vi "Camera.vi"() -> ()   [LabVIEW 2015]
uses:
  Camera Properties.ctl
  ModeEnum.ctl
  CameraState.ctl
  Stack_State.ctl
  Stack Track.ctl
  CameraControlTypeDef.ctl
  Waveform Generation/WaveformControllerState.ctl
  <vilib>/DAQmx/write.llb/DAQmx Write (Digital 1D Wfm NChan NSamp).vi
  <vilib>/DAQmx/write.llb/DAQmx Write (Analog 1D Wfm NChan NSamp).vi
  <vilib>/DAQmx/create/channels.llb/DAQmx Create Channel (AO-Voltage-Basic).vi
  <vilib>/DAQmx/configure/timing.llb/DAQmx Timing (Sample Clock).vi
  <vilib>/Waveform/DWDTOps.llb/DWDT Uncompress Digital.vi
  <vilib>/DAQmx/miscellaneous.llb/DAQmx Fill In Error Info.vi
  <vilib>/DAQmx/create/channels.llb/DAQmx Create Channel (DO-Digital Output).vi
  <vilib>/vision/NI_Vision_Development_Module.lvlib
panel:
  in  "Tab Control":enum32{"Camera Settings", "Recording"}(tab)
  in  "Camera Mode":T1(ring)
  in  "Slit Width /percent":dbl=100.0
  out "error IO":errorcluster
  in  "V Height":dbl=2048.0 min=4.0 max=2048.0 step=4.0
  in  "V Offset":dbl min=0.0 max=0.0 step=4.0
  in  "H Offset":dbl min=0.0 max=0.0 step=4.0
  in  "H Width":dbl min=4.0 max=2048.0 step=4.0
  in  "Exposure /ms":dbl=40.0 min=0.0010036691729323308 max=10.000004210526315 step=1e-08
  in  "Trigger Source":dbl(ring)=2.0 items=["Internal"=1.0, "External"=2.0]
  in  "Readout Direction":dbl(ring)=2.0 items=["Forward"=1.0, "Backward"=2.0]
  in  "Scanning Mode":dbl(ring)=12.0 items=["Full Frame"=1.0, "Slit Scanning"=12.0]
  in  "Advanced DCAM Controls":i32(listbox) caption="Multicolumn Listbox"
  in  "Mode":T2
  in  "FOV /um":dbl(slide) scale=-10.0..10.0
  in  "Properties":T3=4211904 items=["SENSOR MODE"=4212128, "CCD MODE"=4212384, "READOUT MODE"=4211872, "ACTIVE VIEW INDEX"=4343136, "BITS PER CHANNEL"=4342976, "IMAGE PIXEL TYPE"=4343296, "BINNING"=4215968, "EXPOSURE TIME"=2049184, "CONTRAST GAIN"=3163312, "CONTRAST OFFSET"=3163328, "LIGHT MODE"=2114720, "SENSITIVITY"=2114992, "PHOTON IMAGING MODE"=2115200, "HIGH DYNAMIC RANGE MODE"=3163360, "WHITE BALANCE"=3163568, "TEMPERATURE"=2115232, "TEMPERATURE TARGET"=2115264, "SENSOR COOLER FAN"=2115296, "LINEBUNDLE HEIGHT"=4212192, "MECHANICAL SHUTTER"=2115488, "BACK FOCUS POSITION"=8422304, "TRIGGER CONNECTOR"=1066432, "TRIGGER SOURCE"=1066144, "OUTPUT TRIGGER SOURCE"=1852576, "TRIGGER GLOBAL EXPOSURE"=2049680, "FIRST TRIGGER BEHAVIOR"=2049696, "CHANNEL SYNC"=1852352, "READOUT DIRECTION"=4211904, "PRE HSYNC COUNT"=1852704, "INTERNAL LINE SPEED"=4191408, "INTERNAL LINE INVERVAL"=4191424]
  out "Image":T4(plugin-control)
  out "Histogram":T5(graph)
  in  "stop":bool
  in  "Calibration":bool
  in  "MultiD Scan":bool
  in  "Stage Controller":bool
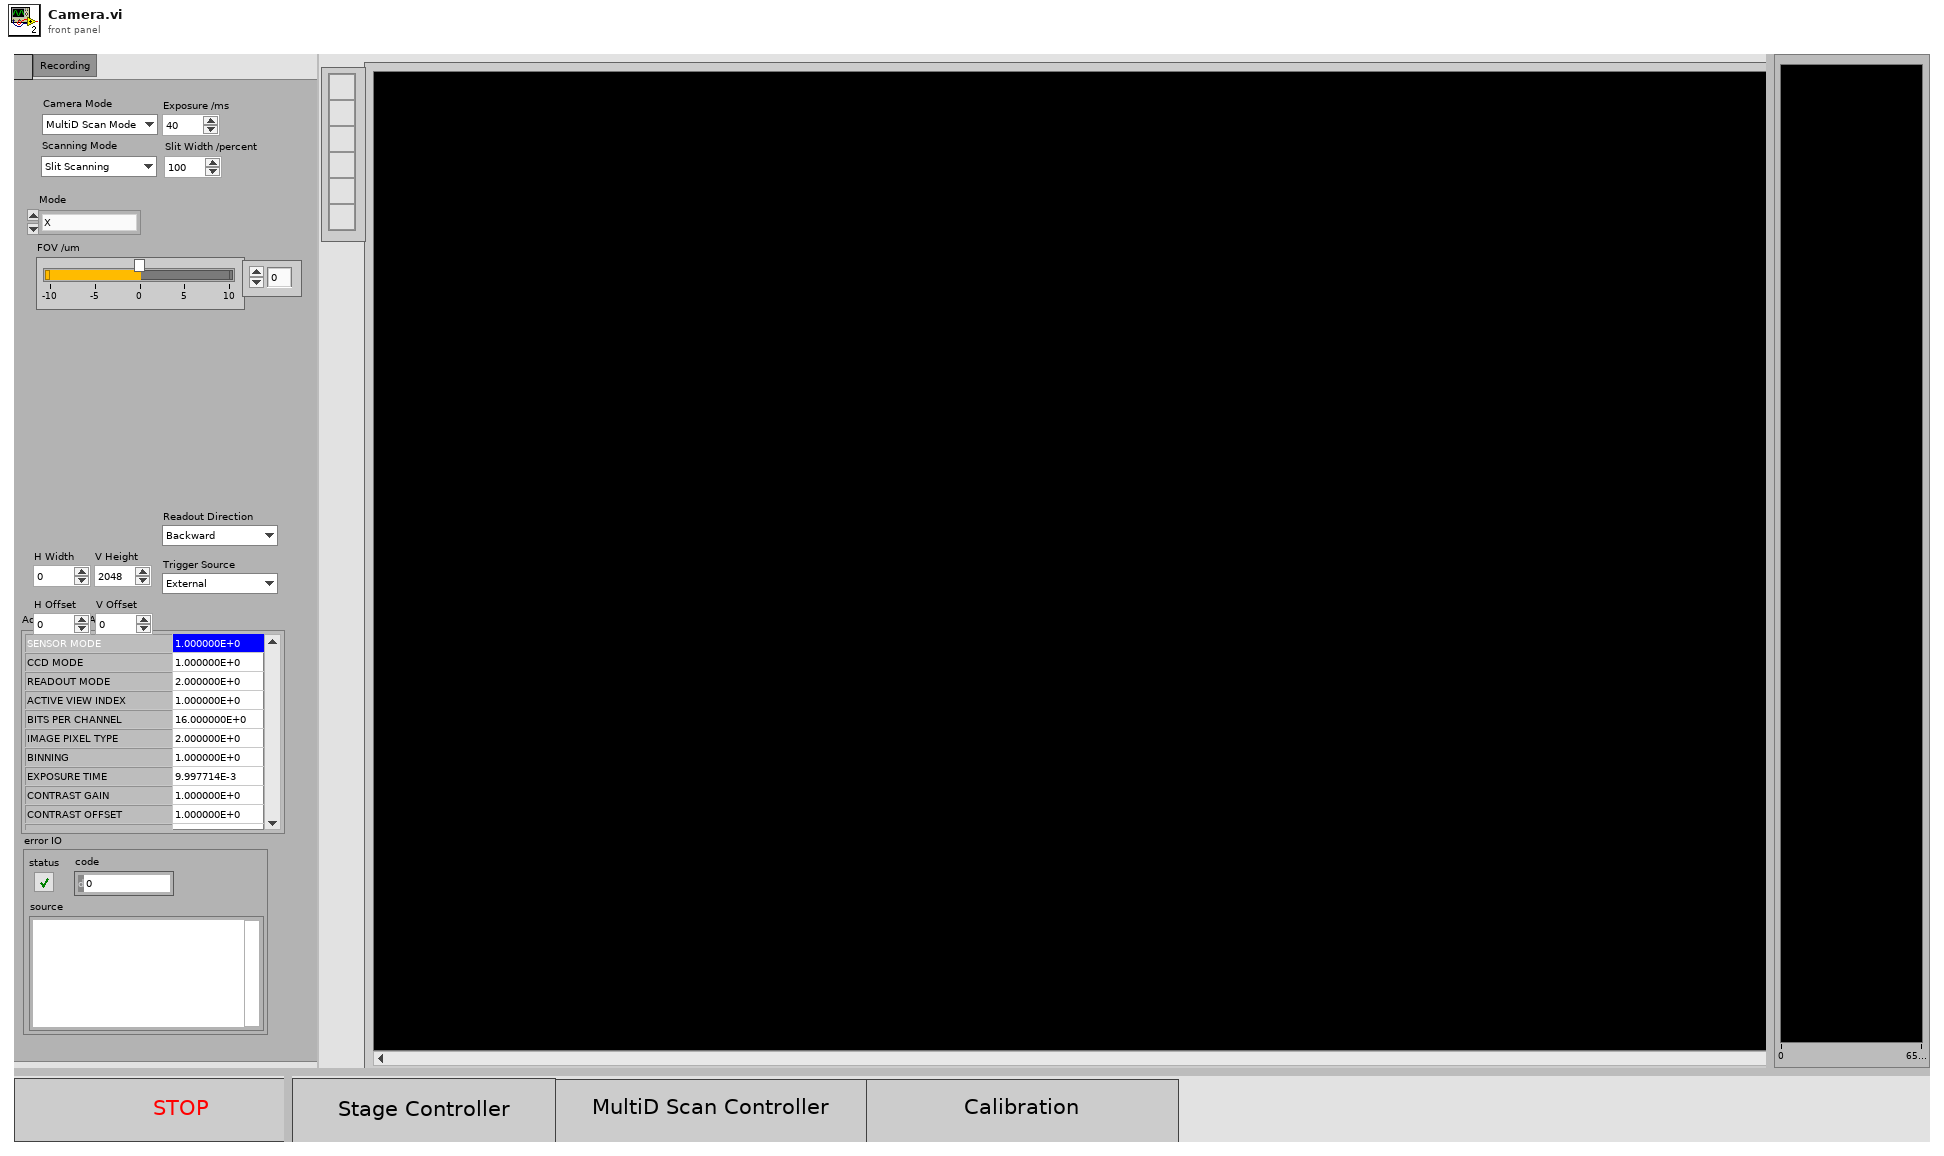
[diagram p1: front panel]
types:
  T1 = enum16{"MultiD Scan Mode", "2D Scan Mode", "Calibration Mode"}
  T2 = typedef "ModeEnum.ctl" = enum16{"X", "XY", "XYZ", "XYZT", "runWaves", "generateWaves", "deInit", "Init", "Idle"}
  T3 = typedef "Camera Properties.ctl" = u32
  T4 = typedef "IMAQ Image.ctl" = refnum<image>
  T5 = cluster{"Starting Value":sgl, "Incremental Value":sgl, "Histogram":u32[]}
  T6 = cluster{"Piezo Position /um":dbl, "Exposure/ms":dbl, "Samples/millisecond":dbl, "Relax/ms":dbl}
  T7 = typedef "WaveformControllerState.ctl" = enum16{"X", "XY", "XYZ", "XYZT", "runWaves", "generateWaves", "deInit", "Init", "Idle"}
  T8 = typedef "CameraControlTypeDef.ctl" = enum16{"IntervalLineInt", "Ram Record", "HardDisk Record", "Disengage Update", "Update", "Idle", "ROI", "Binning", "Scan Mode", "Trigger Mode", "Readout Mode", "Readout Direction", "Preview", "ROIWindow", "Trigger Source"}
  T9 = cluster{"height":u32, "width":u32, "datatype":u32}
  T10 = typedef "Stack_State.ctl" = cluster{"State":T11, "Stack Number":i32, "Image":u16[][], "Stacks":i32}
  T11 = typedef "Stack Track.ctl" = enum16{"Idle", "Display", "Start Sequence", "Read Disk", "STOP", "Collecting", "End"}
  T12 = typedef "CameraState.ctl" = enum16{"init", "active", "deinit"}
  T13 = cluster{T7, cluster{"Piezo Position /um":dbl, "Exposure/ms":dbl, "Samples/millisecond":dbl, "Relax/ms":dbl}}
  T14 = typedef "Image Type" = u32
  T15 = cluster{"Value":i32, "Minimum":i32, "Maximum":i32, "Increment":i32}
  T16 = cluster{"Minimum":i32, "Maximum":i32, "Increment":i32}
  T17 = cluster{"Enum":T8, dbl, "timeout in ms (-1)":u32}
  T18 = cluster{"State":T11, "Timeout":i32, "Data 16":u16[][], "Timeout":i32}
  T19 = cluster{"Enum":T8, "Trigger Source":dbl, "timeout in ms (-1)":i32}
  T20 = cluster{"Enum":T8, "Exposure /ms":dbl, "Parameter":u32}
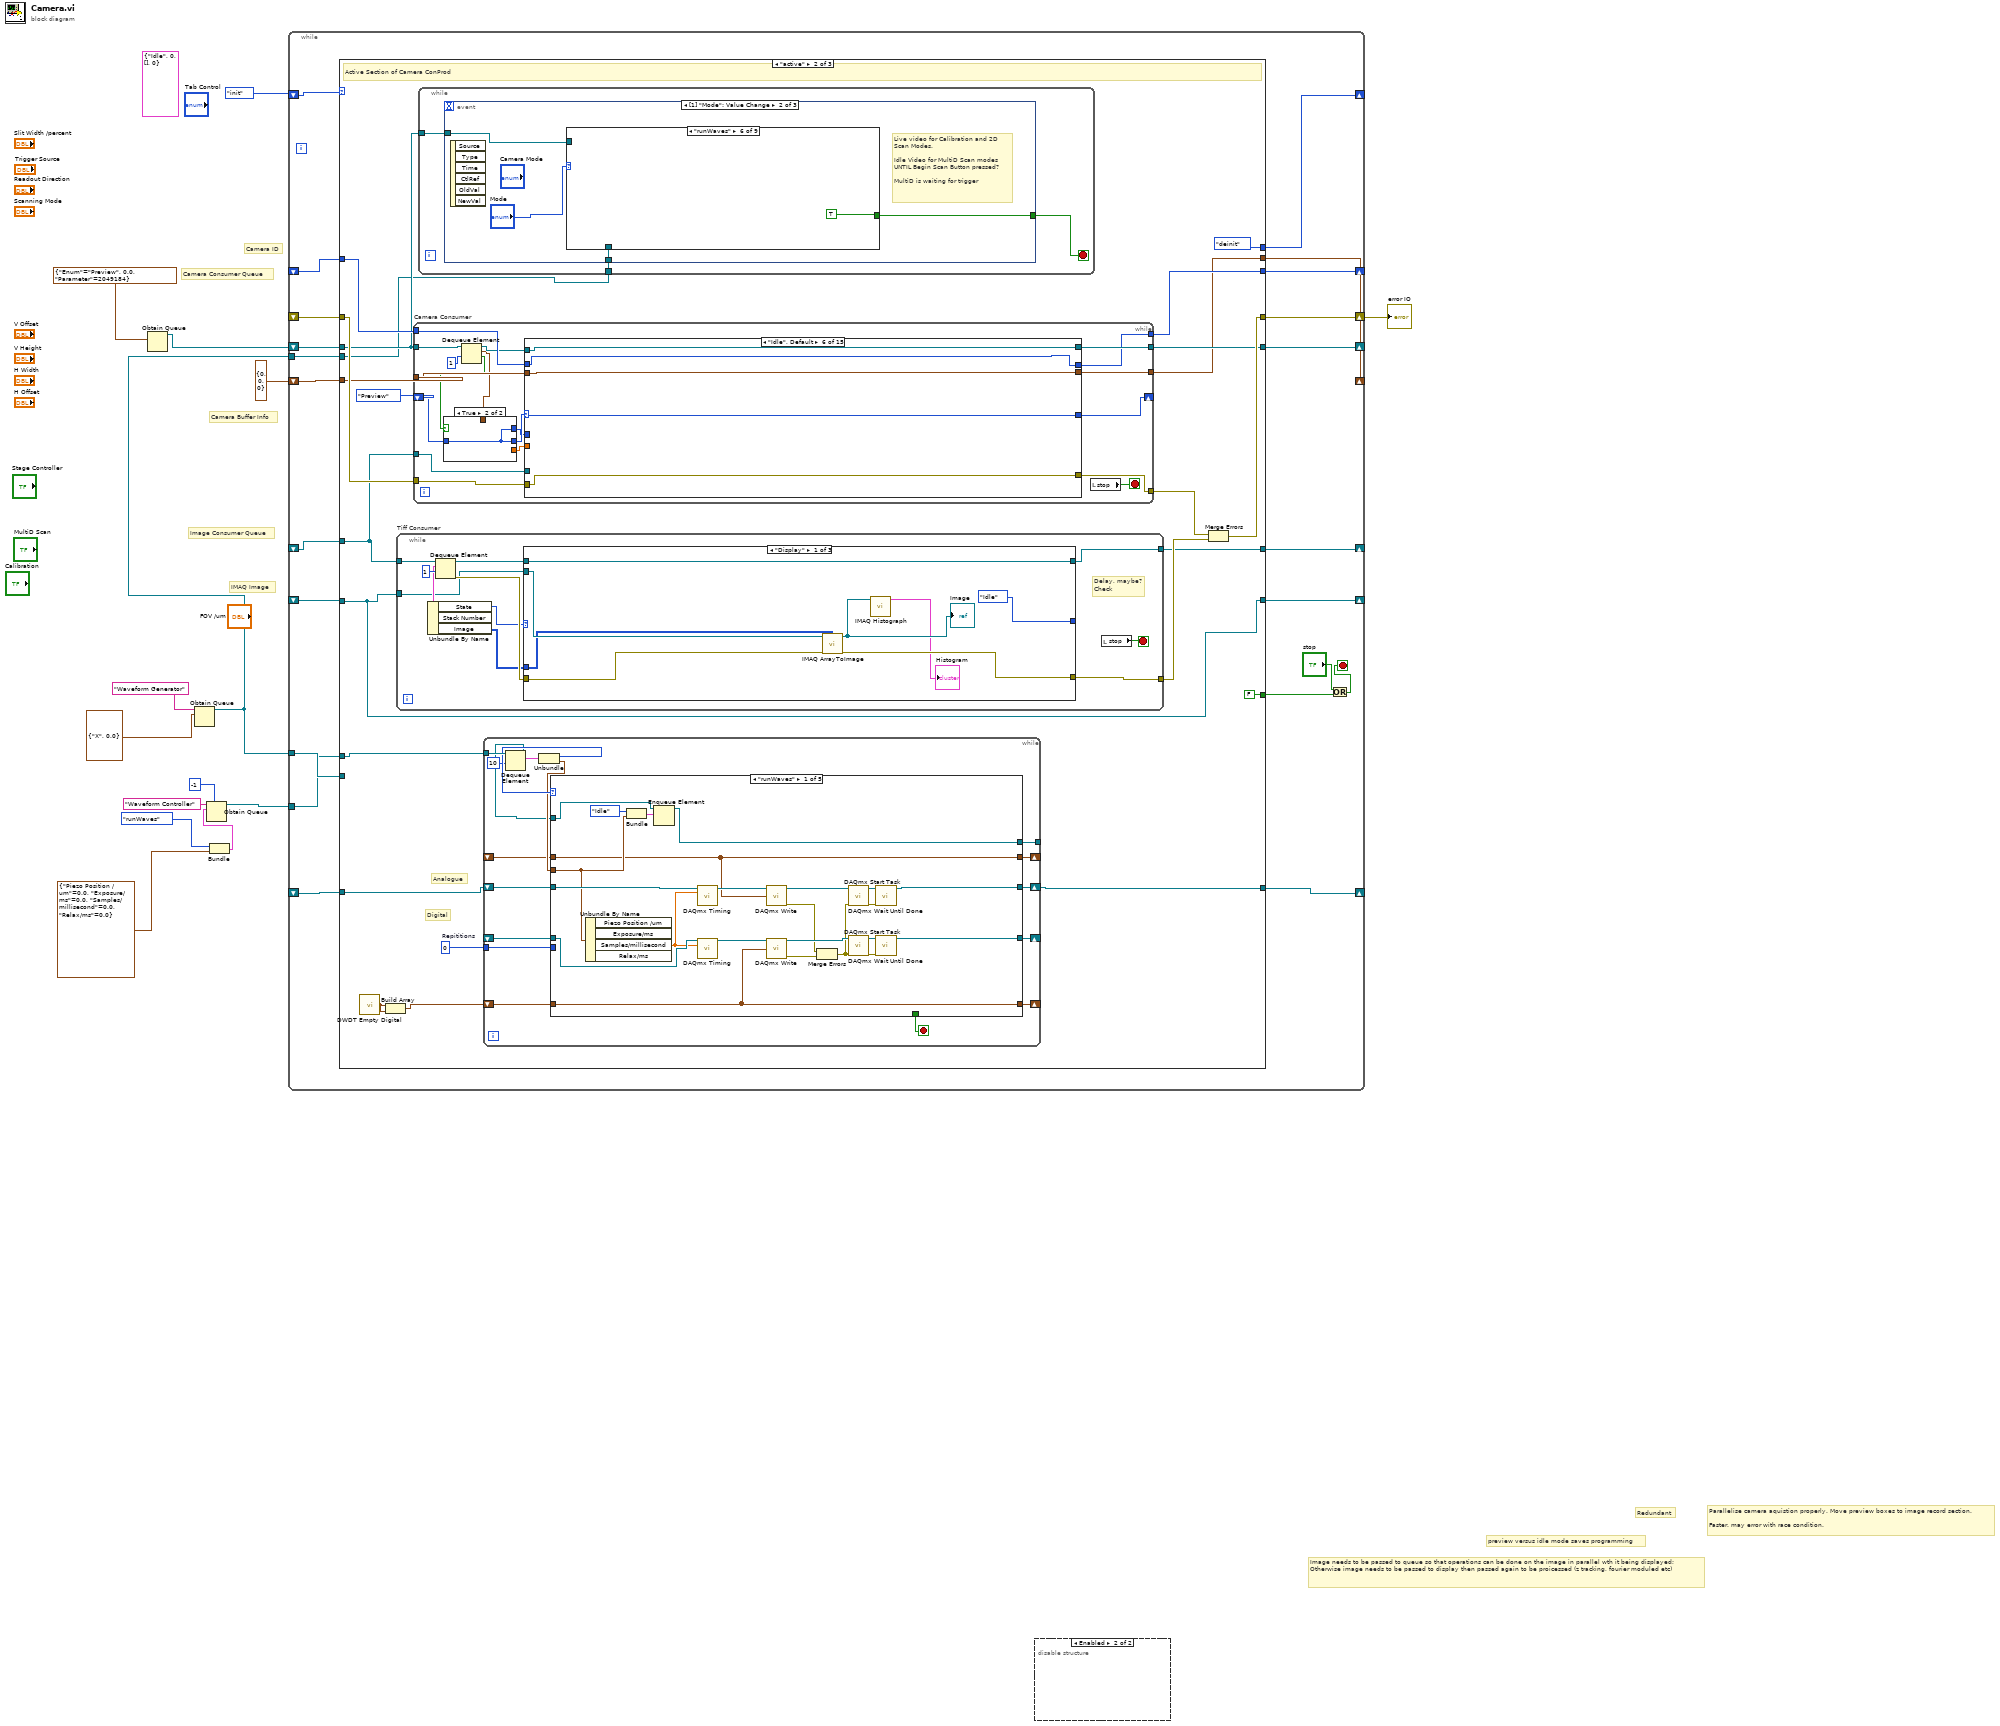
[diagram p0: block diagram]
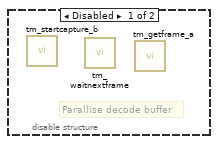
[diagram p2: hidden frame]
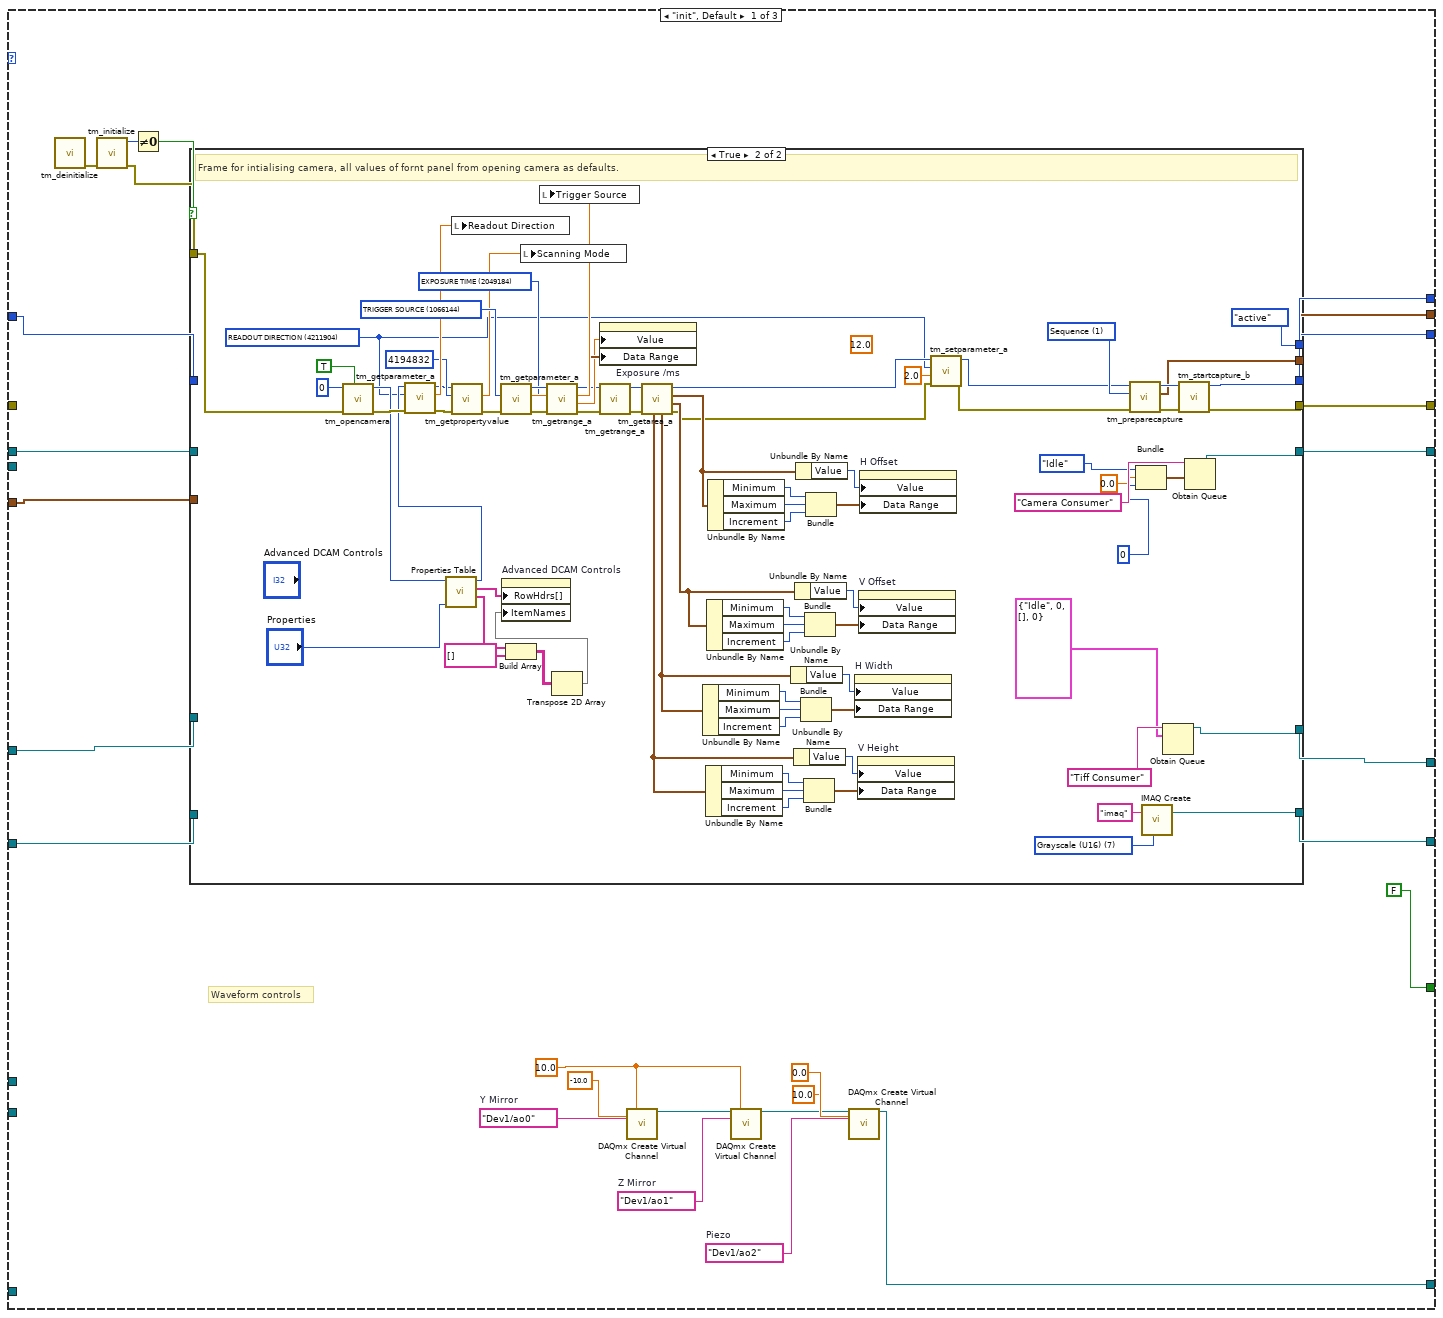
[diagram p3: hidden frame]
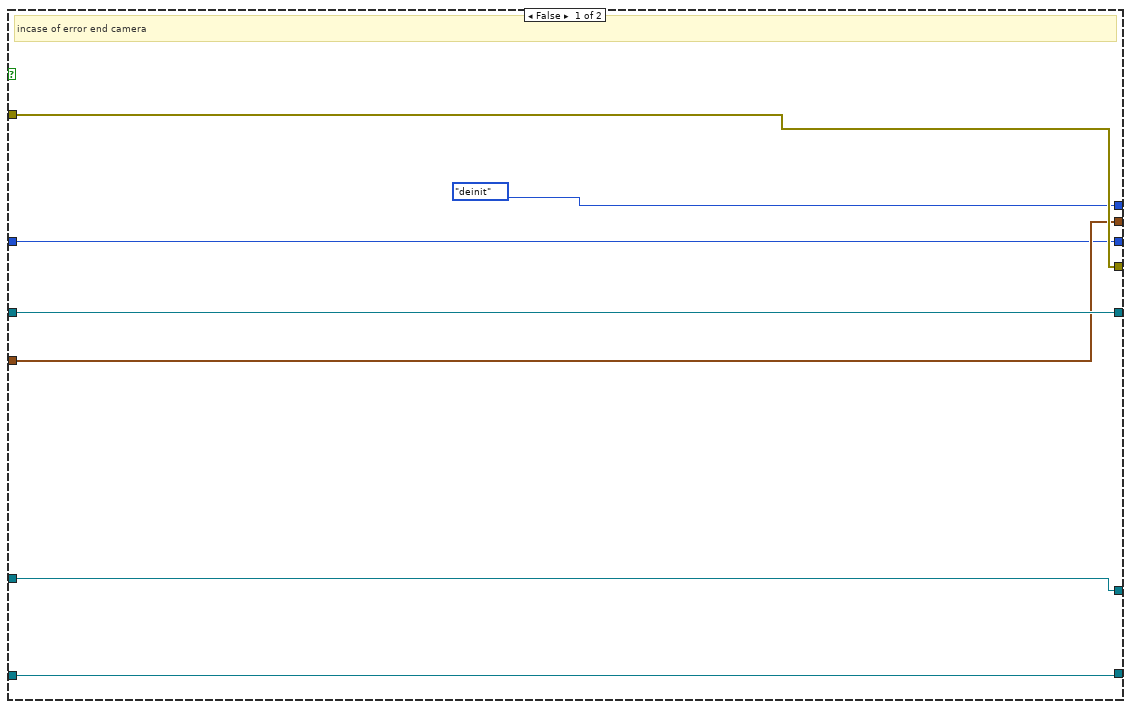
[diagram p4: hidden frame]
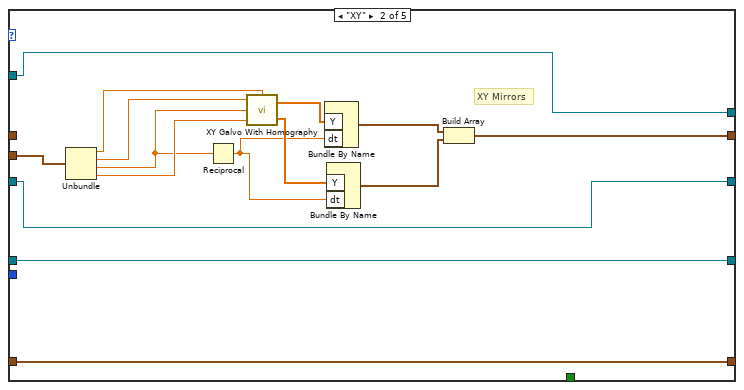
[diagram p5: hidden frame]
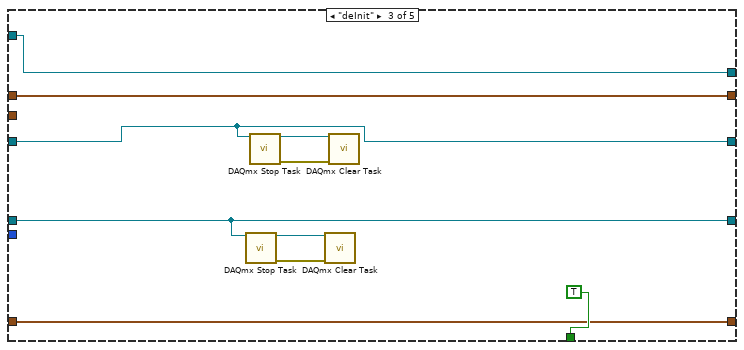
[diagram p6: hidden frame]
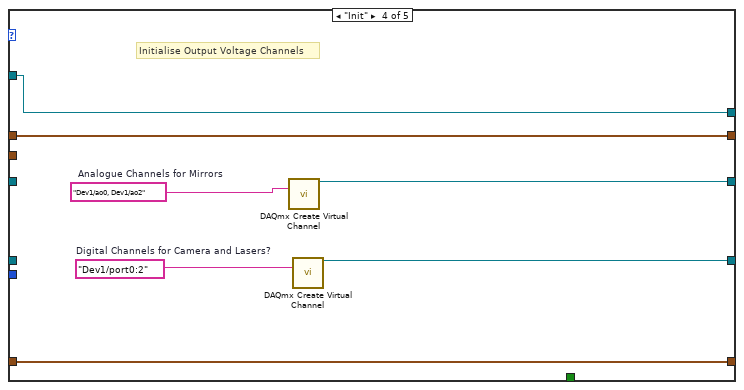
[diagram p7: hidden frame]
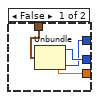
[diagram p11: hidden frame]
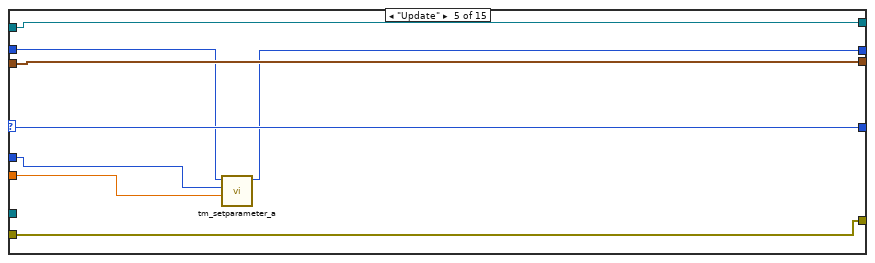
[diagram p16: hidden frame]
diagram:
  (unwired) T10 {"State"=enum."Idle", "Stack Number"=0, "Image"=[], "Stacks"=0} ("input cluster")
  # "IMAQ Image"
  # "Camera Buffer Info"
  # "Image needs to be passed to queue so that operations can be done on the image in parallel wth it being displayed;\nOtherwise image needs to be passed to display then passed again to be proicessed (z tracking, fourier moduled etc)"
  # "preview versus idle mode saves programming"
  # "Parallelise camera aquistion properly. Move preview boxes to image record section.\n\nFaster. may error with race condition."
  # "Redundant"
  # "Image Consumer Queue"
  # "Camera Consumer Queue"
  # "Camera ID"
  n1 = Obtain Queue(element data type=cluster{"Enum":T8, dbl, "Parameter":u32} {"Enum"=enum."Preview", 0.0, "Parameter"=2049184}) -> (queue out=w9:refnum<queue>)  [unwired: 4 in, 2 out]
  n2 = Obtain Queue(name (unnamed)="Waveform Generator", element data type=cluster{"Mode":T2, "Exposure":dbl} {"Mode"=enum."X", "Exposure"=0.0}) -> (queue out=w8:refnum<queue>)  [unwired: 3 in, 2 out]
  n3 = Bundle(WaveformControllerState."runWaves", T6 {"Piezo Position /um"=0.0, "Exposure/ms"=0.0, "Samples/millisecond"=0.0, "Relax/ms"=0.0}) -> (w5:T13)  [unwired: 1 in]
  n4 = Obtain Queue(max queue size (-1, unlimited)=-1, name (unnamed)="Waveform Controller", element data type=w5) -> (queue out=w1:refnum<queue>)  [unwired: 2 in, 2 out]
  n5 = while {
    shift-right: [w36] -> _
    shift-left: CameraState."init" -> [w35]
    shift-right: [w34] -> _
    shift-left: _ -> [w33]
    shift-right: [w32] -> w13
    shift-left: _ -> [w31]
    shift-right: [w29] -> _
    shift-left: _ -> [w28]
    shift-right: [w30] -> _
    shift-left: w9 -> [w27]
    shift-right: [w23] -> _
    shift-left: T9 {"height"=0, "width"=0, "datatype"=0} ("Buffer Info") -> [w22]
    shift-right: [w21] -> _
    shift-left: _ -> [w20]
    tunnel: w8 -> [w19]
    tunnel: w8 -> [w18]
    tunnel: w1 -> [w17]
    shift-right: [w16] -> _
    shift-left: _ -> [w15]
    stop <- w25 stop-if-true
    n6 = case shown="\"active\"" w35 {
      tunnel: [w59 CameraState."deinit" CameraState."init"] -> w36
      tunnel: [w58 w170 w447] -> w34
      tunnel: w33 -> [w49 w171 w447]
      tunnel: [w57 w169 w450] -> w32
      tunnel: w31 -> [_ w163 w451]
      tunnel: [w56 w166 w444] -> w30
      tunnel: [w55 w165 w445] -> w29
      tunnel: w28 -> [w53 w158 w445]
      tunnel: w27 -> [w54 w156 w444]
      tunnel: [FALSE ("stop") FALSE ("stop") TRUE ("stop")] -> w24
      tunnel: [w51 w161 w442] -> w23
      tunnel: w22 -> [w50 w160 w442]
      tunnel: w20 -> [w47 w157 w441]
      tunnel: [w48 w157 w441] -> w21
      tunnel: w19 -> [_ _ _]
      tunnel: w18 -> [_ w155 _]
      tunnel: w17 -> [_ w151 _]
      tunnel: [w37 w149 w440] -> w16
      tunnel: w15 -> [_ w150 w440]
      frame "init", Default {
        w42 = tag "Dev1/ao2"  # Piezo
        w43 = tag "Dev1/ao1"  # Z Mirror
        w44 = tag "Dev1/ao0"  # Y Mirror
        w46 = 10.0 ("maximum value")
        # "Waveform controls"
        n7 = call "tm_deinitialize.vi"() -> ("error out"=w63:errorcluster)  [unwired: 11 in]
        n8 = call "tm_initialize.vi"("error in (no error)"=w63) -> ("error out"=w60:errorcluster, "Number Of Cameras"=w62:u32)  [unwired: 7 in, 2 out]
        n9 = Not Equal To 0?(x=w62) -> (x != 0?=w61:bool)
        n10 = case shown="True" w61 {
          tunnel: w60 -> [w70 w142]
          tunnel: [CameraState."deinit" CameraState."active"] -> w59
          tunnel: [w70 w125] -> w57
          tunnel: [w65 w123] -> w58
          tunnel: [w68 w97] -> w56
          tunnel: [w67 w95] -> w55
          tunnel: w54 -> [w68 _]
          tunnel: w53 -> [w67 _]
          tunnel: [w66 w85] -> w51
          tunnel: w50 -> [w66 _]
          tunnel: w49 -> [w65 _]
          tunnel: [w64 w82] -> w48
          tunnel: w47 -> [w64 _]
          frame False {
            # "incase of error end camera"
          }
          frame True {
            (unwired) 12.0 ("Value in")
            w84 = T14 7 items=["Grayscale (U8)", "Grayscale (I16)", "Grayscale (SGL)", "Complex (CSG)", "RGB (U32)", "HSL (U32)", "RGB (U64)", "Grayscale (U16)"] ("Image Type")
            w127 = 1 items=["Snap", "Sequence"] ("Capture mode")
            w139 = u32 2049184 items=["SENSOR MODE"=4212128, "CCD MODE"=4212384, "READOUT MODE"=4211872, "ACTIVE VIEW INDEX"=4343136, "BITS PER CHANNEL"=4342976, "IMAGE PIXEL TYPE"=4343296, "BINNING"=4215968, "EXPOSURE TIME"=2049184, "CONTRAST GAIN"=3163312, "CONTRAST OFFSET"=3163328, "LIGHT MODE"=2114720, "SENSITIVITY"=2114992, "PHOTON IMAGING MODE"=2115200, "HIGH DYNAMIC RANGE MODE"=3163360, "WHITE BALANCE"=3163568, "TEMPERATURE"=2115232, "TEMPERATURE TARGET"=2115264, "SENSOR COOLER FAN"=2115296, "LINEBUNDLE HEIGHT"=4212192, "MECHANICAL SHUTTER"=2115488, "BACK FOCUS POSITION"=8422304, "TRIGGER CONNECTOR"=1066432, "TRIGGER SOURCE"=1066144, "OUTPUT TRIGGER SOURCE"=1852576, "TRIGGER GLOBAL EXPOSURE"=2049680, "FIRST TRIGGER BEHAVIOR"=2049696, "CHANNEL SYNC"=1852352, "READOUT DIRECTION"=4211904, "PRE HSYNC COUNT"=1852704, "INTERNAL LINE SPEED"=4191408, "INTERNAL LINE INVERVAL"=4191424] ("Parameter")
            w77 = T3 4211904 items=["SENSOR MODE"=4212128, "CCD MODE"=4212384, "READOUT MODE"=4211872, "ACTIVE VIEW INDEX"=4343136, "BITS PER CHANNEL"=4342976, "IMAGE PIXEL TYPE"=4343296, "BINNING"=4215968, "EXPOSURE TIME"=2049184, "CONTRAST GAIN"=3163312, "CONTRAST OFFSET"=3163328, "LIGHT MODE"=2114720, "SENSITIVITY"=2114992, "PHOTON IMAGING MODE"=2115200, "HIGH DYNAMIC RANGE MODE"=3163360, "WHITE BALANCE"=3163568, "TEMPERATURE"=2115232, "TEMPERATURE TARGET"=2115264, "SENSOR COOLER FAN"=2115296, "LINEBUNDLE HEIGHT"=4212192, "MECHANICAL SHUTTER"=2115488, "BACK FOCUS POSITION"=8422304, "TRIGGER CONNECTOR"=1066432, "TRIGGER SOURCE"=1066144, "OUTPUT TRIGGER SOURCE"=1852576, "TRIGGER GLOBAL EXPOSURE"=2049680, "FIRST TRIGGER BEHAVIOR"=2049696, "CHANNEL SYNC"=1852352, "READOUT DIRECTION"=4211904, "PRE HSYNC COUNT"=1852704, "INTERNAL LINE SPEED"=4191408, "INTERNAL LINE INVERVAL"=4191424] ("Parameter")
            w145 = u32 1066144 items=["SENSOR MODE"=4212128, "CCD MODE"=4212384, "READOUT MODE"=4211872, "ACTIVE VIEW INDEX"=4343136, "BITS PER CHANNEL"=4342976, "IMAGE PIXEL TYPE"=4343296, "BINNING"=4215968, "EXPOSURE TIME"=2049184, "CONTRAST GAIN"=3163312, "CONTRAST OFFSET"=3163328, "LIGHT MODE"=2114720, "SENSITIVITY"=2114992, "PHOTON IMAGING MODE"=2115200, "HIGH DYNAMIC RANGE MODE"=3163360, "WHITE BALANCE"=3163568, "TEMPERATURE"=2115232, "TEMPERATURE TARGET"=2115264, "SENSOR COOLER FAN"=2115296, "LINEBUNDLE HEIGHT"=4212192, "MECHANICAL SHUTTER"=2115488, "BACK FOCUS POSITION"=8422304, "TRIGGER CONNECTOR"=1066432, "TRIGGER SOURCE"=1066144, "OUTPUT TRIGGER SOURCE"=1852576, "TRIGGER GLOBAL EXPOSURE"=2049680, "FIRST TRIGGER BEHAVIOR"=2049696, "CHANNEL SYNC"=1852352, "READOUT DIRECTION"=4211904, "PRE HSYNC COUNT"=1852704, "INTERNAL LINE SPEED"=4191408, "INTERNAL LINE INVERVAL"=4191424] ("Parameter")
            # "Frame for intialising camera, all values of fornt panel from opening camera as defaults."
            n11 = call "tm_opencamera.vi"("Force Open"=TRUE, "error in (no error)"=w142, "Camera Index"=u32 0) -> ("error out"=w146:errorcluster, "Handle out"=w93:u32)  [unwired: 6 in, 1 out]
            n12 = call "Properties Table.vi"("Properties"="Properties", "Handle In"=w93) -> ("Value Stirngs Out"=w90:string[], "Row Headers"=w91:string[], "Handle Out"=w92:u32)  [unwired: 3 in, 1 out]
            n13 = call "tm_getparameter_a.vi"("error in (no error)"=w146, "Parameter"=w77, "Handle in"=w92) -> ("error out"=w128:errorcluster, "Value out"=w143:dbl, "Handle out"=w131:u32)  [unwired: 6 in]
            n14 = local write "Readout Direction"(w143) -> ()
            n15 = call "tm_getpropertyvalue.vi"("error in (no error)"=w128, "Property ID"=u32 4194832, "Handle in"=w131) -> ("error out"=w129:errorcluster, "Value in"=w130:sgl)  [unwired: 6 in, 1 out]
            n16 = call "tm_getparameter_a.vi"("error in (no error)"=w129, "Parameter"=w145) -> ("error out"=w140:errorcluster, "Value out"=w144:dbl, "Handle out"=w141:u32)  [unwired: 7 in]
            n17 = Build Array(w90, string[] [] ("element")) -> (w88:string[][])
            n18 = local write "Scanning Mode"(w130) -> ()
            n19 = local write "Trigger Source"(w144) -> ()
            n20 = call "tm_getrange_a.vi"("error in (no error)"=w140, "Parameter"=w139, "Handle in"=w141) -> ("error out"=w135:errorcluster, "default"=w137:dbl, "Range"=w138:cluster{"min":dbl, "max":dbl, "step":dbl}, "Handle out"=w136:u32)  [unwired: 2 in, 3 out]
            n21 = Transpose 2D Array(2D array=w88) -> (transposed array=w87:string[][])
            n22 = property on="Advanced DCAM Controls" class="MCListbox (strict)"("RowHdrs[]"=w91, "ItemNames"=w87) -> ()  [unwired: 2 in, 2 out]
            n23 = property on="Exposure /ms" class="DigNum (strict)"("Value"=w137, "Data Range"=w138) -> ()  [unwired: 2 in, 2 out]
            n24 = call "tm_getrange_a.vi"("error in (no error)"=w135, "Handle in"=w136) -> ("error out"=w134:errorcluster, "Handle out"=w133:u32)  [unwired: 3 in, 5 out]
            n25 = call "tm_getarea_a.vi"("error in (no error)"=w134, "Handle in"=w133) -> ("error out"=w79:errorcluster, "V Offset"=w99:T15, "H Offset"=w122:T15, "Handle out"=w81:u32, "H Width"=w100:T15, "V Width"=w101:T15)  [unwired: 4 in]
            n26 = Unbundle By Name(w100) -> ("Minimum"=w111:i32, "Maximum"=w110:i32, "Increment"=w109:i32)
            n27 = Unbundle By Name(w101) -> ("Minimum"=w102:i32, "Maximum"=w103:i32, "Increment"=w104:i32)
            n28 = Unbundle By Name(w99) -> ("Minimum"=w112:i32, "Maximum"=w113:i32, "Increment"=w114:i32)
            n29 = Unbundle By Name(w122) -> ("Minimum"=w121:i32, "Maximum"=w120:i32, "Increment"=w119:i32)
            n30 = Unbundle By Name(w100) -> ("Value"=w107:i32)
            n31 = Unbundle By Name(w101) -> ("Value"=w106:i32)
            n32 = Unbundle By Name(w99) -> ("Value"=w116:i32)
            n33 = Unbundle By Name(w122) -> ("Value"=w117:i32)
            n34 = Bundle("Minimum"=w111, "Maximum"=w110, "Increment"=w109) -> (w108:T16)  [unwired: 1 in]
            n35 = Bundle("Minimum"=w102, "Maximum"=w103, "Increment"=w104) -> (w105:T16)  [unwired: 1 in]
            n36 = Bundle("Minimum"=w112, "Maximum"=w113, "Increment"=w114) -> (w115:T16)  [unwired: 1 in]
            n37 = Bundle("Minimum"=w121, "Maximum"=w120, "Increment"=w119) -> (w118:T16)  [unwired: 1 in]
            n38 = property on="H Width" class="DigNum (strict)"("Value"=w107, "Data Range"=w108) -> ()  [unwired: 2 in, 2 out]
            n39 = property on="V Height" class="DigNum (strict)"("Value"=w106, "Data Range"=w105) -> ()  [unwired: 2 in, 2 out]
            n40 = property on="V Offset" class="DigNum (strict)"("Value"=w116, "Data Range"=w115) -> ()  [unwired: 2 in, 2 out]
            n41 = property on="H Offset" class="DigNum (strict)"("Value"=w117, "Data Range"=w118) -> ()  [unwired: 2 in, 2 out]
            n42 = call "tm_setparameter_a.vi"("error in (no error)"=w79, "Value in"=2.0, "Parameter"=w77, "Handle in"=w81) -> ("error out"=w78:errorcluster, "Handle out"=w80:u32)  [unwired: 6 in]
            n43 = call "tm_preparecapture.vi"("error in (no error)"=w78, "Capture mode"=w127, "Handle in"=w80) -> ("error out"=w126:errorcluster, "Buffer Info"=w85:T9, "Handle out"=w124:u32)  [unwired: 5 in, 1 out]
            n44 = Bundle("Enum"=CameraControlTypeDef."Idle", 0.0, "timeout in ms (-1)"=u32 0) -> (w73:T17)  [unwired: 1 in]
            n45 = call "IMAQ Create"("Image Name"="imaq", "Image Type"=w84) -> ("New Image"=w82:T4)  [unwired: 3 in, 1 out]
            n46 = Obtain Queue(name (unnamed)="Tiff Consumer", element data type=T10 {"State"=enum."Idle", "Stack Number"=0, "Image"=[], "Stacks"=0} ("input cluster")) -> (queue out=w95:refnum<queue>)  [unwired: 3 in, 2 out]
            n47 = call "tm_startcapture_b.vi"("error in (no error)"=w126, "Handle in"=w124) -> ("error out"=w125:errorcluster, "Handle out"=w123:u32)  [unwired: 8 in]
            n48 = Obtain Queue(name (unnamed)="Camera Consumer", element data type=w73) -> (queue out=w97:refnum<queue>)  [unwired: 3 in, 2 out]
          }
        }
        n49 = call-poly <vilib>:"DAQmx Create Virtual Channel.vi"("maximum value"=w46, "minimum value"=-10.0, "physical channels"=w44) -> ("task out"=w39:refnum<k21>)  [unwired: 11 in, 1 out]
        n50 = call-poly <vilib>:"DAQmx Create Virtual Channel.vi"("task in"=w39, "maximum value"=w46, "physical channels"=w43) -> ("task out"=w38:refnum<k21>)  [unwired: 11 in, 1 out]
        n51 = call-poly <vilib>:"DAQmx Create Virtual Channel.vi"("task in"=w38, "maximum value"=10.0 ("minimum value"), "minimum value"=0.0 ("maximum value"), "physical channels"=w42) -> ("task out"=w37:refnum<k21>)  [unwired: 10 in, 1 out]
      }
      frame "active" {
        w154 = 0  # Repititions
        # "Digital"
        # "Analogue"
        # "Active Section of Camera ConProd"
        n52 = call <vilib>:"DWDT Empty Digital.vi"() -> ("digital waveform out"=w152:digitalwaveform)  [unwired: 5 in]
        n53 = Build Array(w152, w152) -> (w153:digitalwaveform[])
        n54 = while "Tiff Consumer" {
          tunnel: [w252] -> w168
          tunnel: [w255] -> w165
          tunnel: w158 -> [w257]
          tunnel: w157 -> [w249]
          stop <- w259 stop-if-true
          # "Delay, maybe?\nCheck"
          n55 = Dequeue Element(queue=w257, timeout in ms (-1)=1) -> (queue out=w254:refnum<queue>, element=w256:T10, error out=w253:errorcluster)  [unwired: 1 in, 1 out]
          n56 = Unbundle By Name(w256) -> ("State"=w250:T11, "Image"=w251:u16[][])  [unwired: 1 out]
          n57 = case shown="\"Display\"" w250 {
            selector: w250 -> [_ w270 w271]
            tunnel: [w267 w269 w272] -> w255
            tunnel: w254 -> [w267 w269 w272]
            tunnel: [Stack_Track."Idle" ("State") w270 w271] -> _
            tunnel: w251 -> [w262 _ _]
            tunnel: w249 -> [w266 _ _]
            tunnel: w253 -> [w265 w268 w273]
            tunnel: [w264 w268 w273] -> w252
            frame "Display" {
              n58 = call "IMAQ ArrayToImage"("Image Pixels (U16)"=w262, "error in (no error)"=w265, "Image"=w266) -> ("error out"=w264:errorcluster, "Image Out"=w261:T4)  [unwired: 7 in]
              "Image" <- w261
              n59 = call "IMAQ Histograph"("Image"=w261) -> ("Histogram Graph"=→"Histogram":T5)  [unwired: 7 in, 3 out]
            }
            frame "Idle", Default {
            }
            frame "Start Sequence" {
            }
          }
          n60 = local read "stop"() -> (w259:bool)
        }
        n61 = while "Camera Consumer" {
          tunnel: w163 -> [w290]
          tunnel: w171 -> [w287]
          tunnel: [w286] -> w170
          tunnel: [w289] -> w167
          tunnel: w156 -> [w282]
          tunnel: [w291] -> w166
          shift-right: [w288] -> _
          shift-left: CameraControlTypeDef."Preview" ("Enum") -> [w278]
          tunnel: [w285] -> w161
          tunnel: w160 -> [w284]
          tunnel: w158 -> [w277]
          stop <- w292 stop-if-true
          n62 = Dequeue Element(queue=w282, timeout in ms (-1)=1) -> (queue out=w281:refnum<queue>, element=w276:cluster{"Enum":T8, dbl, "Parameter":u32}, timed out?=w280:bool)  [unwired: 1 in, 1 out]
          n63 = case shown="True" w280 {
            tunnel: [w295 w297] -> w279
            tunnel: w278 -> [_ w297]
            tunnel: w276 -> [w296 _]
            tunnel: [w294 _] -> w275
            tunnel: [w293 w297] -> w274
            frame False {
              n64 = Unbundle(w296) -> ("Enum"=w295:T8, w294:dbl, "Parameter"=w293:u32)
            }
            frame True {
            }
          }
          n65 = case shown="\"Idle\", Default" w279 {
            selector: w279 -> [w301 w306 w311 w316 w324 w329 w334 w339 w344 w349 w354 w359 _ w378 _]
            tunnel: w281 -> [w300 w307 w312 w317 w325 w330 w335 w340 w345 w350 w355 w360 w375 w380 w385]
            tunnel: [w300 w307 w312 w317 w325 w330 w335 w340 w345 w350 w355 w360 w375 w380 w385] -> w291
            tunnel: w290 -> [w302 w305 w310 w315 w323 w328 w333 w338 w343 w348 w353 w358 w365 w377 w383]
            tunnel: [w302 w305 w310 w315 w323 w328 w333 w338 w343 w348 w353 w358 w369 w377 w383] -> w289
            tunnel: [w301 w306 w311 w316 w324 w329 w334 w339 w344 w349 w354 w359 CameraControlTypeDef."Preview" ("Enum") w378 CameraControlTypeDef."Preview" ("Enum")] -> w288
            tunnel: w287 -> [w299 w304 w309 w314 w321 w327 w332 w337 w342 w347 w352 w357 w373 w379 w384]
            tunnel: [w299 w304 w309 w314 w320 w327 w332 w337 w342 w347 w352 w357 w371 w379 w384] -> w286
            tunnel: [w298 w303 w308 w313 w322 w326 w331 w336 w341 w346 w351 w356 w367 w376 w382] -> w285
            tunnel: w284 -> [w298 w303 w308 w313 w322 w326 w331 w336 w341 w346 w351 w356 w367 w376 w382]
            tunnel: w277 -> [_ _ _ _ _ _ _ _ _ _ _ _ w366 _ _]
            tunnel: w275 -> [_ _ _ _ w318 _ _ _ _ _ _ _ _ _ _]
            tunnel: w274 -> [_ _ _ _ w319 _ _ _ _ _ _ _ _ _ _]
            frame "IntervalLineInt" {
            }
            frame "Ram Record" {
            }
            frame "HardDisk Record" {
            }
            frame "Disengage Update" {
            }
            frame "Update" {
              n66 = call "tm_setparameter_a.vi"("Value in"=w318, "Parameter"=w319, "Handle in"=w321) -> ("Handle out"=w320:u32)  [unwired: 7 in, 1 out]
            }
            frame "Idle", Default {
            }
            frame "ROI" {
            }
            frame "Binning" {
            }
            frame "Scan Mode" {
            }
            frame "Trigger Mode" {
            }
            frame "Readout Mode" {
            }
            frame "Readout Direction" {
            }
            frame "Preview" {
              w362 = 0 ("Timeout")
              n67 = call "tm_waitnextframe.vi"("error in (no error)"=w365, "Timeout"=3000, "Handle in"=w373) -> ("error out"=w370:errorcluster, "Handle out"=w372:u32)  [unwired: 5 in, 2 out]
              n68 = call "tm_getframe_a.vi"("error in (no error)"=w370, "Buffer Info"=w367, "Handle in"=w372) -> ("error out"=w369:errorcluster, "Data 16"=w363:u16[][], "Handle out"=w371:u32)  [unwired: 4 in, 2 out]
              n69 = Bundle("State"=Stack_Track."Display", "Timeout"=w362, "Data 16"=w363, "Timeout"=w362) -> (w361:T18)  [unwired: 1 in]
              n70 = Enqueue Element(queue=w366, element=w361, error in (no error)=w365) -> ()  [unwired: 1 in, 3 out]
            }
            frame "ROIWindow" {
            }
            frame "Trigger Source" {
              n71 = call "tm_unpreparecapture.vi"() -> ()  [unwired: 10 in, 2 out]
              n72 = call "tm_setparameter_a.vi"() -> ()  [unwired: 10 in, 2 out]
              n73 = call "tm_preparecapture.vi"() -> ()  [unwired: 8 in, 4 out]
            }
          }
          n74 = local read "stop"() -> (w292:bool)
        }
        n75 = while {
          tunnel: w156 -> [w387]
          tunnel: w155 -> [w386]
          stop <- w388 stop-if-true
          n76 = event shown="[1] \"Mode\": Value Change" {
            selector: _ -> [_ _ _]
            dyn-events: _ -> [_ _ _]
            timeout: _ -> [_ _ _]
            tunnel: [w389 w390 _] -> w388
            tunnel: w387 -> [_ w393 w438]
            tunnel: w386 -> [_ w391 w435]
            event "stop": Value Change {
              n77 = event-data() -> ()  [unwired: 1 in, 6 out]
              n78 = local read "stop"() -> (w389:bool)
            }
            event Value Change {
              # "Live video for Calibration and 2D\nScan Modes.\n\nIdle Video for MultiD Scan modes\nUNTIL Begin Scan Button pressed?\n\nMultiD is waiting for trigger"
              n79 = event-data() -> ()  [unwired: 1 in, 6 out]
              n80 = case shown="\"runWaves\"" "Mode" {
                selector: "Mode" -> [w396 _ _ _ w419 _ _ _ _]
                tunnel: w393 -> [w404 w412 _ _ w428 _ _ _ _]
                tunnel: w391 -> [w397 _ w415 _ w418 _ _ _ _]
                tunnel: [_ _ _ _ _ TRUE FALSE _ _] -> w390
                frame "X" {
                  w398 = 0 ("timeout in ms (-1)")
                  w399 = 1.0 items=["Internal"=1.0, "External"=2.0] ("Trigger Source")
                  n81 = Bundle("Enum"=CameraControlTypeDef."Readout Mode", "Trigger Source"=w399, "timeout in ms (-1)"=w398) -> (w403:T19)  [unwired: 1 in]
                  n82 = Enqueue Element(queue=w404, element=w403) -> (queue out=w401:refnum<queue>)  [unwired: 2 in, 2 out]
                  n83 = Bundle("Enum"=CameraControlTypeDef."Preview", "Trigger Source"=w399, "timeout in ms (-1)"=w398) -> (w402:T19)  [unwired: 1 in]
                  n84 = Bundle("Mode"=w396, "Exposure /ms"=0.0) -> (w395:cluster{"Mode":T2, "Exposure /ms":dbl})  [unwired: 1 in]
                  n85 = Enqueue Element(queue=w401, element=w402) -> ()  [unwired: 2 in, 3 out]
                  n86 = Enqueue Element(queue=w397, element=w395) -> ()  [unwired: 2 in, 3 out]
                }
                frame "XYZ" {
                  w406 = 0 ("timeout in ms (-1)")
                  w407 = 2.0 items=["Internal"=1.0, "External"=2.0] ("Trigger Source")
                  n87 = Bundle("Enum"=CameraControlTypeDef."Readout Mode", "Trigger Source"=w407, "timeout in ms (-1)"=w406) -> (w411:T19)  [unwired: 1 in]
                  n88 = Enqueue Element(queue=w412, element=w411) -> (queue out=w410:refnum<queue>)  [unwired: 2 in, 2 out]
                  n89 = Bundle("Enum"=CameraControlTypeDef."Idle", "Trigger Source"=w407, "timeout in ms (-1)"=w406) -> (w409:T19)  [unwired: 1 in]
                  n90 = Enqueue Element(queue=w410, element=w409) -> ()  [unwired: 2 in, 3 out]
                }
                frame "generateWaves" {
                  w417 = ModeEnum."generateWaves"  # Mode
                  n91 = local read "Exposure /ms"() -> (w416:dbl)
                  n92 = Bundle("Mode"=w417, "Exposure /ms"=w416) -> (w414:cluster{"Mode":T2, "Exposure /ms":dbl})  [unwired: 1 in]
                  n93 = Enqueue Element(queue=w415, element=w414) -> ()  [unwired: 2 in, 3 out]
                }
                frame "XYZT" {
                }
                frame "XY" {
                  w422 = 0 ("timeout in ms (-1)")
                  w423 = 2.0 items=["Internal"=1.0, "External"=2.0] ("Trigger Source")
                  n94 = local read "Exposure /ms"() -> (w420:dbl)
                  n95 = Bundle("Enum"=CameraControlTypeDef."Readout Mode", "Trigger Source"=w423, "timeout in ms (-1)"=w422) -> (w427:T19)  [unwired: 1 in]
                  n96 = Enqueue Element(queue=w428, element=w427) -> (queue out=w424:refnum<queue>)  [unwired: 2 in, 2 out]
                  n97 = Bundle("Mode"=w419, "Exposure /ms"=w420) -> (w421:cluster{"Mode":T2, "Exposure /ms":dbl})  [unwired: 1 in]
                  n98 = Bundle("Enum"=CameraControlTypeDef."Preview", "Trigger Source"=w423, "timeout in ms (-1)"=w422) -> (w426:T19)  [unwired: 1 in]
                  n99 = Enqueue Element(queue=w418, element=w421) -> ()  [unwired: 2 in, 3 out]
                  n100 = Enqueue Element(queue=w424, element=w426) -> ()  [unwired: 2 in, 3 out]
                }
                frame "runWaves" {
                }
                frame "deInit" {
                }
                frame "Init" {
                }
                frame "Idle" {
                }
              }
            }
            event "Exposure /ms": Value Change {
              w434 = ModeEnum."generateWaves"  # Mode
              w436 = u32 2049184 items=["SENSOR MODE"=4212128, "CCD MODE"=4212384, "READOUT MODE"=4211872, "ACTIVE VIEW INDEX"=4343136, "BITS PER CHANNEL"=4342976, "IMAGE PIXEL TYPE"=4343296, "BINNING"=4215968, "EXPOSURE TIME"=2049184, "CONTRAST GAIN"=3163312, "CONTRAST OFFSET"=3163328, "LIGHT MODE"=2114720, "SENSITIVITY"=2114992, "PHOTON IMAGING MODE"=2115200, "HIGH DYNAMIC RANGE MODE"=3163360, "WHITE BALANCE"=3163568, "TEMPERATURE"=2115232, "TEMPERATURE TARGET"=2115264, "SENSOR COOLER FAN"=2115296, "LINEBUNDLE HEIGHT"=4212192, "MECHANICAL SHUTTER"=2115488, "BACK FOCUS POSITION"=8422304, "TRIGGER CONNECTOR"=1066432, "TRIGGER SOURCE"=1066144, "OUTPUT TRIGGER SOURCE"=1852576, "TRIGGER GLOBAL EXPOSURE"=2049680, "FIRST TRIGGER BEHAVIOR"=2049696, "CHANNEL SYNC"=1852352, "READOUT DIRECTION"=4211904, "PRE HSYNC COUNT"=1852704, "INTERNAL LINE SPEED"=4191408, "INTERNAL LINE INTERVAL"=4191424] ("Parameter")
              n101 = event-data() -> ()  [unwired: 1 in, 6 out]
              n102 = Bundle("Enum"=CameraControlTypeDef."Update", "Exposure /ms"="Exposure /ms", "Parameter"=w436) -> (w437:T20)  [unwired: 1 in]
              n103 = Enqueue Element(queue=w438, element=w437) -> ()  [unwired: 2 in, 3 out]
              n104 = Bundle("Mode"=w434, "Exposure /ms"="Exposure /ms") -> (w432:cluster{"Mode":T2, "Exposure /ms":dbl})  [unwired: 1 in]
              n105 = Enqueue Element(queue=w435, element=w432) -> ()  [unwired: 2 in, 3 out]
            }
          }
        }
        n106 = while {
          tunnel: w151 -> [w188]
          shift-right: [w183] -> _
          shift-left: _ -> [w182]
          tunnel: w154 -> [w181]
          tunnel: [w179] -> _
          shift-right: [w177] -> w149
          shift-left: w150 -> [w175]
          shift-right: [w178] -> _
          shift-left: _ -> [w176]
          shift-right: [w174] -> _
          shift-left: w153 -> [w173]
          stop <- w187 stop-if-true
          n107 = Dequeue Element(queue=w188, timeout in ms (-1)=10) -> (queue out=w180:refnum<queue>, element=w186:T13)  [unwired: 1 in, 2 out]
          n108 = Unbundle(w186) -> (w185:T7, w184:T6)
          n109 = case shown="\"runWaves\"" w185 {
            tunnel: [_ _ TRUE _ _] -> w187
            tunnel: w184 -> [w206 w226 _ _ _]
            tunnel: [w201 w216 w234 w243 w247] -> w183
            tunnel: w182 -> [w201 _ w234 w243 w247]
            tunnel: w181 -> [_ _ _ _ _]
            tunnel: w180 -> [w211 w215 w235 w242 w248]
            tunnel: [w210 w215 w235 w242 w248] -> w179
            tunnel: [w191 w213 w228 w239 w246] -> w178
            tunnel: [w193 w214 w227 w238 w245] -> w177
            tunnel: w176 -> [w205 w213 w228 _ w246]
            tunnel: w175 -> [w207 w214 w227 _ w245]
            tunnel: [w200 w212 w233 w237 w244] -> w174
            tunnel: w173 -> [w200 w212 w233 w237 w244]
            frame "runWaves" {
              n110 = Unbundle By Name(w206) -> ("Samples/millisecond"=w204:dbl)  [unwired: 3 out]
              n111 = Bundle(WaveformControllerState."Idle", w206) -> (w208:T13)  [unwired: 1 in]
              n112 = Enqueue Element(queue=w211, element=w208) -> (queue out=w210:refnum<queue>)  [unwired: 2 in, 2 out]
              n113 = call-poly <vilib>:"DAQmx Timing.vi"("task/channels in"=w207, "rate"=w204) -> ("task out"=w203:refnum<k21>)  [unwired: 12 in, 1 out]
              n114 = call-poly <vilib>:"DAQmx Timing.vi"("task/channels in"=w205, "rate"=w204) -> ("task out"=w202:refnum<k21>)  [unwired: 12 in, 1 out]
              n115 = call-poly <vilib>:"DAQmx Write.vi"("task/channels in"=w203, "data"=w201) -> ("task out"=w199:refnum<k21>, "error out"=w196:errorcluster)  [unwired: 11 in, 1 out]
              n116 = call-poly <vilib>:"DAQmx Write.vi"("task/channels in"=w202, "data"=w200) -> ("task out"=w198:refnum<k21>, "error out"=w197:errorcluster)  [unwired: 11 in, 1 out]
              n117 = Merge Errors(w196, w197) -> (w195:errorcluster)
              n118 = call <vilib>:"DAQmx Start Task.vi"("task/channels in"=w199, "error in"=w195) -> ("task out"=w194:refnum<k21>, "error out"=w189:errorcluster)  [unwired: 12 in]
              n119 = call <vilib>:"DAQmx Start Task.vi"("task/channels in"=w198, "error in"=w195) -> ("task out"=w192:refnum<k21>, "error out"=w190:errorcluster)  [unwired: 12 in]
              n120 = call <vilib>:"DAQmx Wait Until Done.vi"("task/channels in"=w194, "error in"=w189) -> ("task out"=w193:refnum<k21>)  [unwired: 12 in, 1 out]
              n121 = call <vilib>:"DAQmx Wait Until Done.vi"("task/channels in"=w192, "error in"=w190) -> ("task out"=w191:refnum<k21>)  [unwired: 12 in, 1 out]
            }
            frame "XY" {
              # "XY Mirrors"
              n122 = Unbundle(w226) -> ("Piezo Position /um"=w225:dbl, "Exposure/ms"=w224:dbl, "Samples/millisecond"=w221:dbl, "Relax/ms"=w223:dbl)
              n123 = Reciprocal(x=w221) -> (1/x=w219:dbl)
              n124 = call "XY Galvo With Homography.vi"("Piezo Position (um)"=w225, "Relax (ms)"=w223, "Samples /Millisecond"=w221, "Exposure (ms)"=w224) -> ("Z Mirror Signal"=w220:dbl[], "Scan Mirror Signal"=w222:dbl[])
              n125 = Bundle By Name("Y"=w222, "dt"=w219) -> (w217:waveform(dbl))  [unwired: 1 in]
              n126 = Bundle By Name("Y"=w220, "dt"=w219) -> (w218:waveform(dbl))  [unwired: 1 in]
              n127 = Build Array(w217, w218) -> (w216:waveform(dbl)[])
            }
            frame "deInit" {
              n128 = call <vilib>:"DAQmx Stop Task.vi"("task/channels in"=w228) -> ("task out"=w229:refnum<k21>, "error out"=w230:errorcluster)  [unwired: 13 in]
              n129 = call <vilib>:"DAQmx Stop Task.vi"("task/channels in"=w227) -> ("task out"=w232:refnum<k21>, "error out"=w231:errorcluster)  [unwired: 13 in]
              n130 = call <vilib>:"DAQmx Clear Task.vi"("task in"=w229, "error in"=w230) -> ()  [unwired: 13 in, 1 out]
              n131 = call <vilib>:"DAQmx Clear Task.vi"("task in"=w232, "error in"=w231) -> ()  [unwired: 13 in, 1 out]
            }
            frame "Init" {
              w240 = tag "Dev1/port0:2"  # Digital Channels for Camera and Lasers?
              w241 = tag "Dev1/ao0, Dev1/ao2"  # Analogue Channels for Mirrors
              # "Initialise Output Voltage Channels"
              n132 = call-poly <vilib>:"DAQmx Create Virtual Channel.vi"("physical channels"=w241) -> ("task out"=w238:refnum<k21>)  [unwired: 13 in, 1 out]
              n133 = call-poly <vilib>:"DAQmx Create Virtual Channel.vi"("lines"=w240) -> ("task out"=w239:refnum<k21>)  [unwired: 13 in, 1 out]
            }
            frame "Idle", Default {
            }
          }
        }
        n134 = Merge Errors(w167, w168) -> (w169:errorcluster)
      }
      frame "deinit" {
        n135 = call "tm_stopcapture.vi"("error in (no error)"=w451, "Handle in"=w447) -> ("error out"=w454:errorcluster, "Handle out"=w453:u32)  [unwired: 8 in]
        n136 = call "tm_unpreparecapture.vi"("error in (no error)"=w454, "Handle in"=w453) -> ("error out"=w455:errorcluster, "Handle out"=w452:u32)  [unwired: 8 in]
        n137 = call "tm_closecamera.vi"("error in (no error)"=w455, "Handle in"=w452) -> ("error out"=w456:errorcluster)  [unwired: 9 in]
        n138 = call "tm_deinitialize.vi"("error in (no error)"=w456) -> ("error out"=w457:errorcluster)  [unwired: 10 in]
        n139 = Release Queue(queue=w445, error in (no error)=w457) -> (error out=w449:errorcluster)  [unwired: 1 in, 2 out]
        n140 = Release Queue(queue=w444, error in (no error)=w457) -> (error out=w448:errorcluster)  [unwired: 1 in, 2 out]
        n141 = Merge Errors(w449, w448) -> (w450:errorcluster)
      }
    }
    n142 = Or(x="stop", y=w24) -> (x .or. y?=w25:bool)
  }
  "error IO" <- w13
  n143 = disable-structure shown="Enabled" {
    frame Disabled {
      # "Parallise decode buffer"
      n144 = call "tm_startcapture_b.vi"() -> ()  [unwired: 10 in, 2 out]
      n145 = call "tm_waitnextframe.vi"() -> ()  [unwired: 8 in, 4 out]
      n146 = call "tm_getframe_a.vi"() -> ()  [unwired: 7 in, 5 out]
    }
    frame Enabled {
    }
  }
